vi "00 - Calling Python.vi"() -> ()   [LabVIEW 2026]
uses:
  <vilib>/Utility/sysdir.llb/System Directory Type.ctl
  <vilib>/numeric/Random Number (Range) U64.vi
  <vilib>/numeric/sub_Random U32.vi
panel:
  out "Array":u32[](array[colorbox])
  out "Colormap Map":map{string, u32[]}(c390)
  out "Colormap Names":string[](array[string])
  out "Intensity Graph 2":dbl[][](graph)
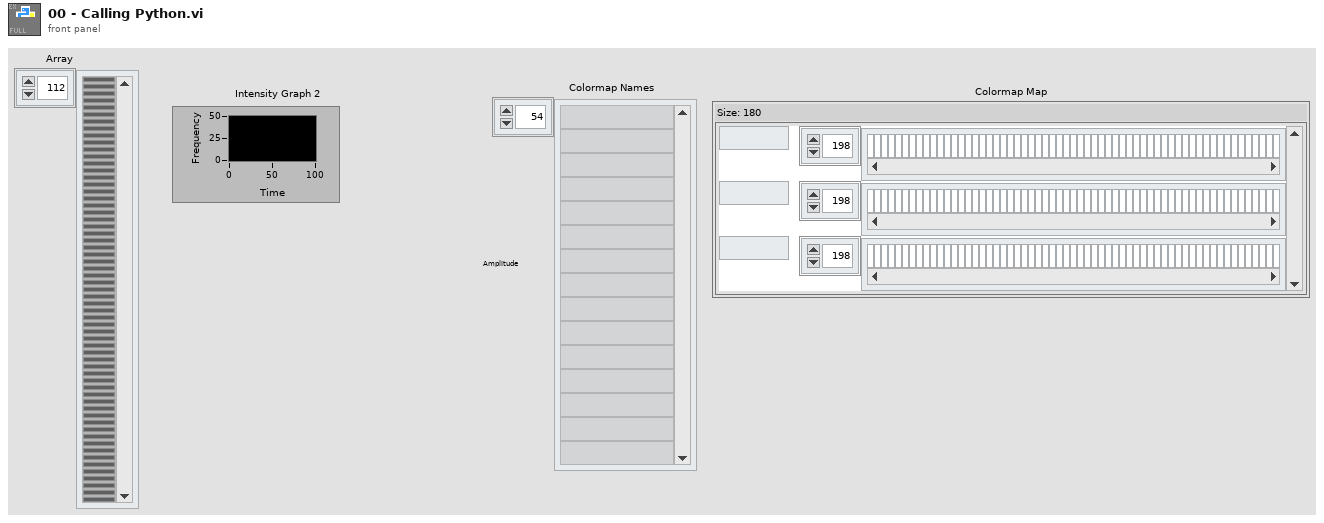
[diagram p1: front panel]
types:
  T1 = enum16{"open", "replace", "create", "open or create", "replace or create", "replace or create with confirmation"}
  T2 = typedef "System Directory Type.ctl" = i32
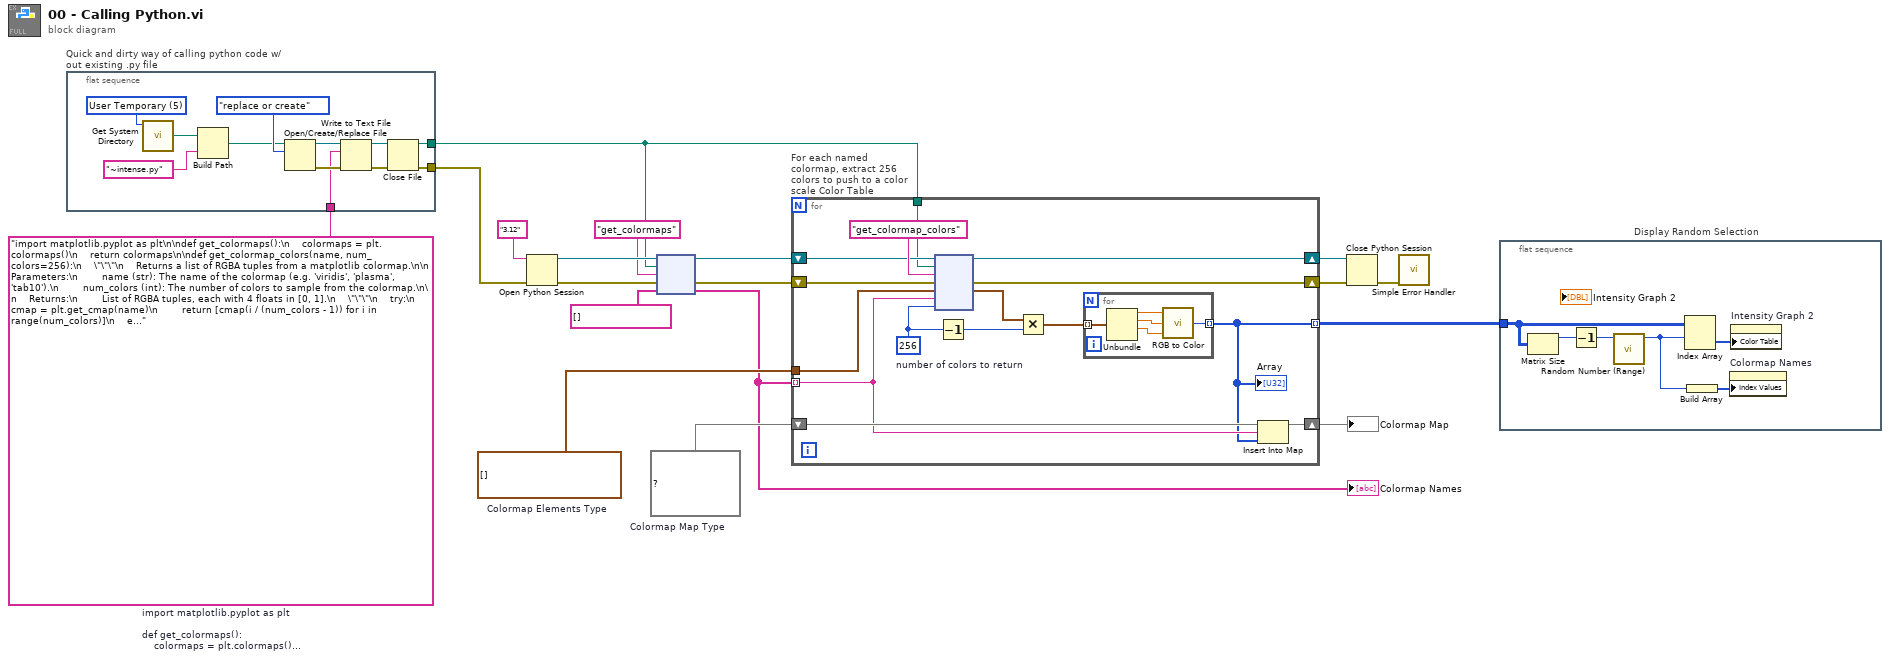
[diagram p0: block diagram]
diagram:
  w4 = cluster{"R":dbl, "G":dbl, "B":dbl, "A":dbl}[] []  # Colormap Elements Type
  w10 = map{string, u32[]} {}  # Colormap Map Type
  w5 = "import matplotlib.pyplot as plt\n\ndef get_colormaps():\n    colormaps = plt.colormaps()\n    return colormaps\n\ndef get_colormap_colors(name, num_colors=256):\n    \"\"\"\n    Returns a list of RGBA tuples from a matplotlib colormap.\n\n    Parameters:\n        name (str): The name of the colormap (e.g. 'viridis', 'plasma', 'tab10').\n        num_colors (int): The number of colors to sample from the colormap.\n\n    Returns:\n        List of RGBA tuples, each with 4 floats in [0, 1].\n    \"\"\"\n    try:\n        cmap = plt.get_cmap(name)\n        return [cmap(i / (num_colors - 1)) for i in range(num_colors)]\n    except ValueError:\n        raise ValueError(f\"Colormap '{name}' not found in matplotlib.\")"  # import matplotlib.pyplot as plt  def get_colormaps():     colormaps = plt.colormaps()     return colormaps  def get_colormap_colors(name, num_colors=256):     """     Returns a list of RGBA tuples from a matplotlib colormap.      Parameters:         name (str): The name of the colormap (e.g. 'viridis', 'plasma', 'tab10').         num_colors (int): The number of colors to sample from the colormap.      Returns:         List of RGBA tuples, each with 4 floats in [0, 1].     """     try:         cmap = plt.get_cmap(name)         return [cmap(i / (num_colors - 1)) for i in range(num_colors)]     except ValueError:         raise ValueError(f"Colormap '{name}' not found in matplotlib.")
  n1 = flat-sequence "Quick and dirty way of calling python code w/out existing .py file" {
    tunnel: [w28] -> w17
    tunnel: [w23] -> w13
    tunnel: w5 -> [w21]
    frame #0 {
      w22 = T2 5 items=["User Home"=0, "User Desktop"=1, "User Documents"=2, "User Application Data"=3, "User Preferences"=4, "User Temporary"=5, "Public Documents"=6, "Public Application Data"=7, "Public Preferences"=8, "Public Cache"=13, "System Core Libraries"=9, "System Installed Libraries"=10, "Application Files"=11, "Boot Volume Root"=12] ("system directory type")
      n2 = call <vilib>:"Get System Directory.vi"("system directory type"=w22) -> ("system directory"=w24:path)  [unwired: 10 in]
      n3 = Build Path(base path=w24, name or relative path="~intense.py") -> (appended path=w19:path)
      n4 = Open/Create/Replace File(file path (use dialog)=w19, operation (0:open)=T1."replace or create") -> (refnum out=w27:refnum<file>, error out=w26:errorcluster)  [unwired: 4 in, 1 out]
      n5 = Write to Text File(file (use dialog)=w27, text=w21, error in=w26) -> (refnum out=w29:refnum<file>, error out=w30:errorcluster)  [unwired: 1 in, 1 out]
      n6 = Close File(refnum=w29, error in=w30) -> (path=w23:path, error out=w28:errorcluster)
    }
  }
  n7 = Open Python Session(python version="3.12" ("Python version"), 3:w17) -> (session out=w15:refnum<k35>, error out=w18:errorcluster)  [unwired: 1 in]
  n8 = node(w15, w13, "get_colormaps" ("function name"), w18, string[] [] ("function name")) -> (w14:refnum<k35>, w16:errorcluster, w3:string[])  [unwired: 2 out]
  "Colormap Names" <- w3
  n9 = for "For each named colormap, extract 256 colors to push to a color scale Color Table" {
    tunnel: [w31] -> w2 mode=indexing
    tunnel: w13 -> [w39]
    tunnel: w3 -> [w34] mode=indexing
    shift-right: [w38] -> w7
    shift-left: w10 -> [w37]
    tunnel: w4 -> [w45]
    shift-right: [w35] -> w8
    shift-left: w16 -> [w41]
    shift-right: [w36] -> w9
    shift-left: w14 -> [w40]
    w32 = 256  # number of colors to return
    n10 = node(w40, w39, "get_colormap_colors" ("function name"), w41, w45, w34, w32) -> (w36:refnum<k35>, w35:errorcluster, w43:cluster{"R":dbl, "G":dbl, "B":dbl, "A":dbl}[])  [unwired: 2 in, 2 out]
    n11 = Decrement(x=w32) -> (x-1=w33:i32)
    n12 = Multiply(x=w43, y=w33) -> (x*y=w42:cluster{"R":dbl, "G":dbl, "B":dbl, "A":dbl}[])
    n13 = for {
      tunnel: w42 -> [w50] mode=indexing
      tunnel: [w46] -> w31 mode=indexing
      n14 = Unbundle(w50) -> ("R"=w49:dbl, "G"=w48:dbl, "B"=w47:dbl)  [unwired: 1 out]
      n15 = call <vilib>:"RGB to Color.vi"("B"=w47, "G"=w48, "R"=w49) -> ("Color"=w46:u32)
    }
    "Array" <- w31
    n16 = Insert Into Map(map in=w37, key=w34, value=w31) -> (map out=w38:map{string, u32[]})  [unwired: 2 out]
  }
  "Colormap Map" <- w7
  n17 = Close Python Session(session in=w9, error in=w8) -> (11:w1:errorcluster)
  n18 = call <vilib>:"Simple Error Handler.vi"("error in (no error)"=w1) -> ()  [unwired: 4 in, 5 out]
  n19 = flat-sequence "Display Random Selection" {
    tunnel: w2 -> [w56]
    frame #0 {
      n20 = Matrix Size(0:w56) -> (1:w55:i32)  [unwired: 1 out]
      n21 = Decrement(x=w55) -> (x-1=w54:i32)
      n22 = call-poly <vilib>:"Random Number (Range).vi"("upper bound (100)"=w54) -> ("number"=w53:u64)  [unwired: 10 in]
      n23 = Index Array(array=w56, index (row)=w53) -> (element=w51:u32[])  [unwired: 1 in]
      n24 = Build Array(w53) -> (w52:u64[])
      n25 = property on="Colormap Names" class="Arr (strict)"("Index Values"=w52) -> ()  [unwired: 2 in, 2 out]
      n26 = property on="Intensity Graph 2" class="IntGraph (strict)"("Color Table"=w51) -> ()  [unwired: 2 in, 2 out]
    }
  }
